vi "Example Callback.vi"() -> ()   [LabVIEW 2013]
uses:
  C:/tf/play/labview/Tinkerforge.dll
panel:
  out "altitude (m)":sgl format="%#_13g"
  in  "stop":bool
  out "air pressure (mbar)":sgl format="%#_13g"
  in  "uid":string="jmQ"
  in  "port":i32=4223
  in  "host":string="localhost"
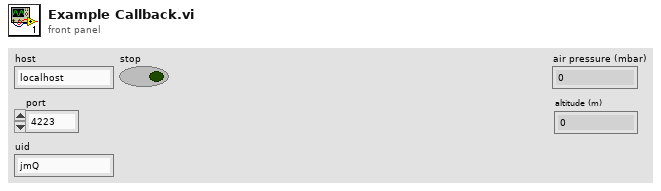
[diagram p1: front panel]
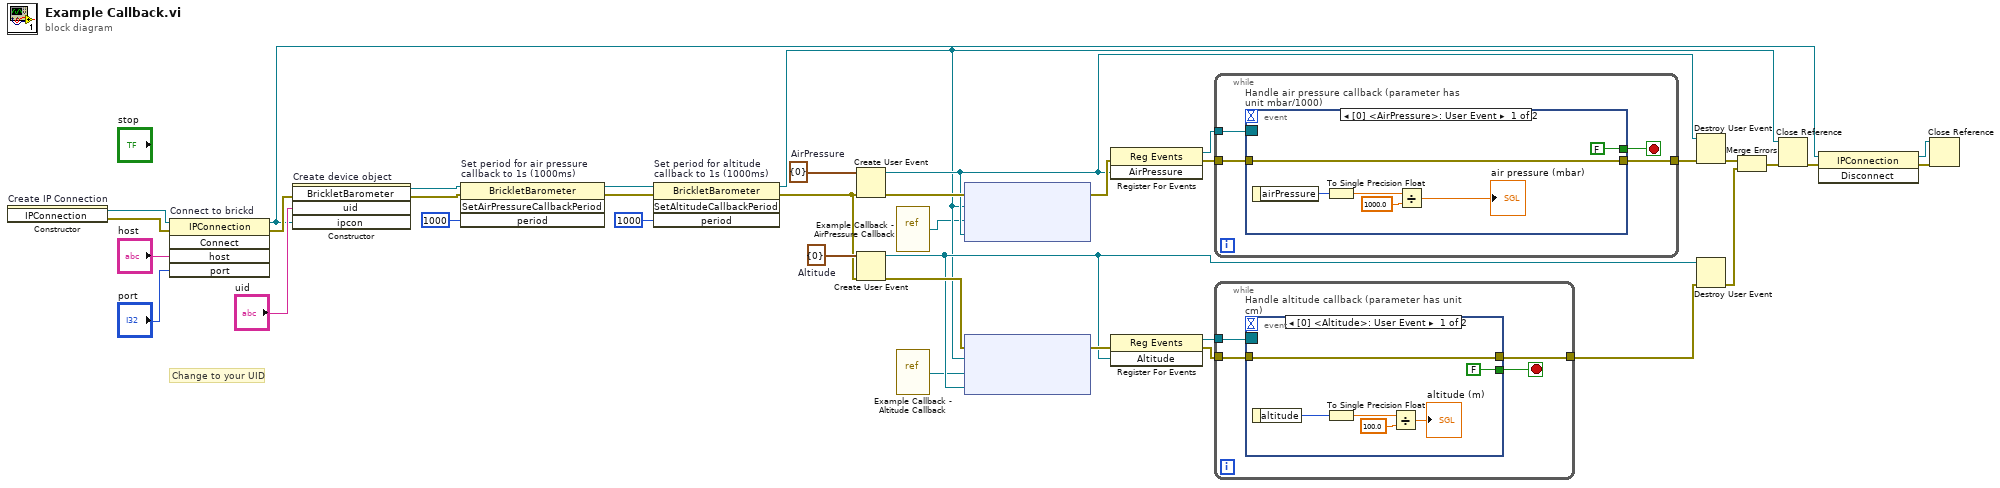
[diagram p0: block diagram]
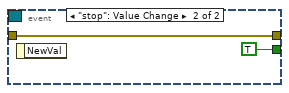
[diagram p2: hidden frame]
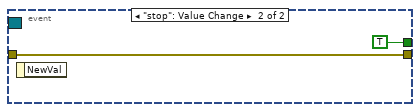
[diagram p3: hidden frame]
diagram:
  w13 = cluster{"altitude":i32} {"altitude"=0}  # Altitude
  w22 = cluster{"airPressure":i32} {"airPressure"=0}  # AirPressure
  # "Change to your UID"
  n1 = constructor on="Create IP Connection" class="IPConnection"() -> (reference out=w37:refnum<k24>, error out=w1:errorcluster)  [unwired: 3 in, 1 out]
  n2 = invoke on="Connect to brickd" class="IPConnection" method="Connect"(reference=w37, error in=w1, "host"="host", "port"="port") -> (reference out=w30:refnum<k24>, error out=w33:errorcluster)  [unwired: 1 in, 3 out]
  n3 = constructor on="Create device object" class="BrickletBarometer"(error in=w33, "uid"="uid", "ipcon"=w30) -> (reference out=w4:refnum<k24>, error out=w7:errorcluster)  [unwired: 2 in, 3 out]
  n4 = invoke on="Set period for air pressure\ncallback to 1s (1000ms)" class="BrickletBarometer" method="SetAirPressureCallbackPeriod"(reference=w4, error in=w7, "period"=i64 1000) -> (reference out=w5:refnum<k24>, error out=w6:errorcluster)  [unwired: 1 in, 2 out]
  n5 = invoke on="Set period for altitude\ncallback to 1s (1000ms)" class="BrickletBarometer" method="SetAltitudeCallbackPeriod"(reference=w5, error in=w6, "period"=i64 1000) -> (reference out=w14:refnum<k24>, error out=w12:errorcluster)  [unwired: 1 in, 2 out]
  n6 = Create User Event(user event datatype=w22, error in=w12) -> (user event=w23:refnum<user-event>, error out=w28:errorcluster)
  n7 = Create User Event(user event datatype=w13, error in=w12) -> (user event=w15:refnum<user-event>, error out=w20:errorcluster)
  n8 = vi-ref "Example Callback - AirPressure Callback.vi"() -> ("vi reference"=w3:refnum<vi>)
  n9 = vi-ref "Example Callback - Altitude Callback.vi"() -> ("vi reference"=w2:refnum<vi>)
  n10 = node ("Register Event Callback")(w28, w14, w3, w23) -> (w27:errorcluster)  [unwired: 1 in, 1 out]
  n11 = node ("Register Event Callback")(w20, w14, w2, w15) -> (w19:errorcluster)  [unwired: 1 in, 1 out]
  n12 = register-events(error in=w27, w23) -> (reference out=w26:refnum<event-registration>, error out=w24:errorcluster)  [unwired: 1 in]
  n13 = register-events(error in=w19, w15) -> (reference out=w18:refnum<event-registration>, error out=w16:errorcluster)  [unwired: 1 in]
  n14 = while {
    tunnel: w26 -> [w41]
    tunnel: [w40] -> w25
    tunnel: w24 -> [w39]
    stop <- w38 stop-if-true
    n15 = event "Handle air pressure callback (parameter has unit mbar/1000)" shown="[0] <AirPressure>: User Event" {
      selector: w41 -> [_ _]
      dyn-events: _ -> [_ _]
      timeout: _ -> [_ _]
      tunnel: [w44 w48] -> w40
      tunnel: w39 -> [w44 w48]
      tunnel: [FALSE TRUE] -> w38
      event User Event {
        n16 = event-data() -> ("airPressure"=w45:i32)  [unwired: 1 in]
        n17 = To Single Precision Float(number=w45) -> (single precision float=w46:sgl)
        n18 = Divide(x=w46, y=sgl 1000.0) -> (x/y=→"air pressure (mbar)":sgl)
      }
      event "stop": Value Change {
        n19 = event-data() -> ()  [unwired: 1 in, 1 out]
      }
    }
  }
  n20 = while {
    tunnel: w18 -> [w53]
    tunnel: [w52] -> w17
    tunnel: w16 -> [w51]
    stop <- w50 stop-if-true
    n21 = event "Handle altitude callback (parameter has unit cm)" shown="[0] <Altitude>: User Event" {
      selector: w53 -> [_ _]
      dyn-events: _ -> [_ _]
      timeout: _ -> [_ _]
      tunnel: [w56 w60] -> w52
      tunnel: w51 -> [w56 w60]
      tunnel: [FALSE TRUE] -> w50
      event User Event {
        n22 = event-data() -> ("altitude"=w57:i32)  [unwired: 1 in]
        n23 = To Single Precision Float(number=w57) -> (single precision float=w58:sgl)
        n24 = Divide(x=w58, y=sgl 100.0) -> (x/y=→"altitude (m)":sgl)
      }
      event "stop": Value Change {
        n25 = event-data() -> ()  [unwired: 1 in, 1 out]
      }
    }
  }
  n26 = Destroy User Event(user event=w23, error in=w25) -> (error out=w10:errorcluster)
  n27 = Destroy User Event(user event=w15, error in=w17) -> (error out=w11:errorcluster)
  n28 = Merge Errors(w10, w11) -> (w9:errorcluster)
  n29 = Close Reference(reference=w14, error in (no error)=w9) -> (error out=w32:errorcluster)
  n30 = invoke class="IPConnection" method="Disconnect"(reference=w30, error in=w32) -> (reference out=w29:refnum<k24>, error out=w31:errorcluster)  [unwired: 1 in, 1 out]
  n31 = Close Reference(reference=w29, error in (no error)=w31) -> ()  [unwired: 1 out]
